vi "db_test.vi"() -> ()   [LabVIEW 2011]
uses:
  <vilib>/addons/database/Connection.llb/DB Tools Open Connec (String).vi
  <vilib>/addons/database/Auxilliary.llb/DB Tools Format Datetime String (Time Stamp).vi
  <vilib>/addons/database/NI_Database_API.lvlib
panel:
  out "output cluster":T1
  in  "sensor1":dbl
  in  "sensor0":dbl
  in  "angle":dbl
  out "date/time string":string
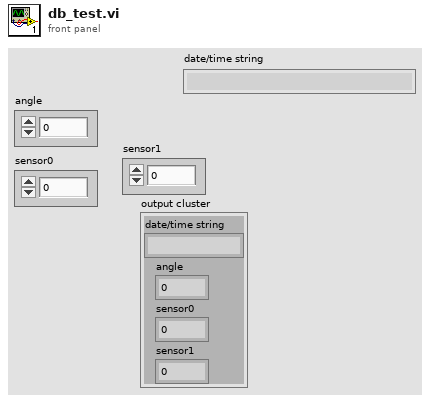
[diagram p1: front panel]
types:
  T1 = cluster{"date/time string":string, "angle":dbl, "sensor0":dbl, "sensor1":dbl}
  T2 = typedef "NI_Database_API.lvlib/Conn ObjectReference.ctl" = refnum<k1>
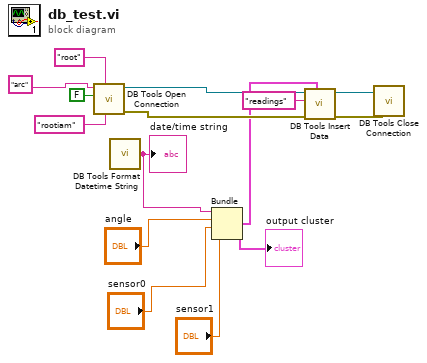
[diagram p0: block diagram]
diagram:
  n1 = call-poly <vilib>:"DB Tools Open Connection.vi"("password"="rootiam", "userID"="root", "prompt? (F)"=FALSE, "connection information"="arc") -> ("error out"=w11:errorcluster, "connection reference"=w12:T2)  [unwired: 4 in]
  n2 = call-poly <vilib>:"DB Tools Format Datetime String.vi"() -> ("date/time string"=w2:string)  [unwired: 1 in]
  "date/time string" <- w2
  n3 = Bundle("date/time string"=w2, "angle"="angle", "sensor0"="sensor0", "sensor1"="sensor1") -> (w1:T1)  [unwired: 1 in]
  "output cluster" <- w1
  n4 = call <vilib>:"DB Tools Insert Data.vi"("data"=w1, "error in (no error)"=w11, "table"="readings", "connection reference"=w12) -> ("error out"=w13:errorcluster, "connection reference out"=w14:T2)  [unwired: 6 in]
  n5 = call <vilib>:"DB Tools Close Connection.vi"("error in (no error)"=w13, "connection reference"=w14) -> ()  [unwired: 5 in, 1 out]
